vi "Add Module To Project.vi"(6 "TreeControl in":refnum<vi>, 7 "Data Cluster In":T1, 8 "error in":errorcluster) -> (0 "error out":errorcluster, 5 "Data Cluster Out":T1={"DQMH Scan Results"={"All DQMH Modules Refs"=[], "All Modules Descriptions"=[], "All Modules type"=[], "Project References"={"Project Ref"=refnum, "Project Name"="", "App Ref"=refnum, "Target"=refnum, "Target Name"=""}, "Dependencies"=[]}, "Current Selection"={"VI Ref"=refnum, "DQMH Lib Ref"=refnum}, "Module type"=enum."Singleton", "Module ID"=-1, "Theme"=FALSE, "Broadcast?"=FALSE, "Tree Selection"="", "Tree Map"={}})   [LabVIEW 2019, in "Panther Dashboard.lvlib"]
doc: "Gets the Singleton and Cloneable references and creates a list of each type of DQMH Modules"
uses:
  Panther Dashboard.lvlib
  Module Data--cluster.ctl
  DQMH Modules Info--cluster.ctl
  Module type--enum.ctl
  Project References--cluster.ctl
  <vilib>/National Instruments/Tree Map/Tree Map Data.ctl
  <vilib>/National Instruments/Tree Map/API/List Roots.vi
  <vilib>/National Instruments/Tree Map/Utility/Into Tree Control Items.vi
  <vilib>/Delacor/Delacor QMH/Libraries/Scripting API/DQMH_Scripting API.lvlib
  <vilib>/National Instruments/Tree Map/Tree Map.lvlib
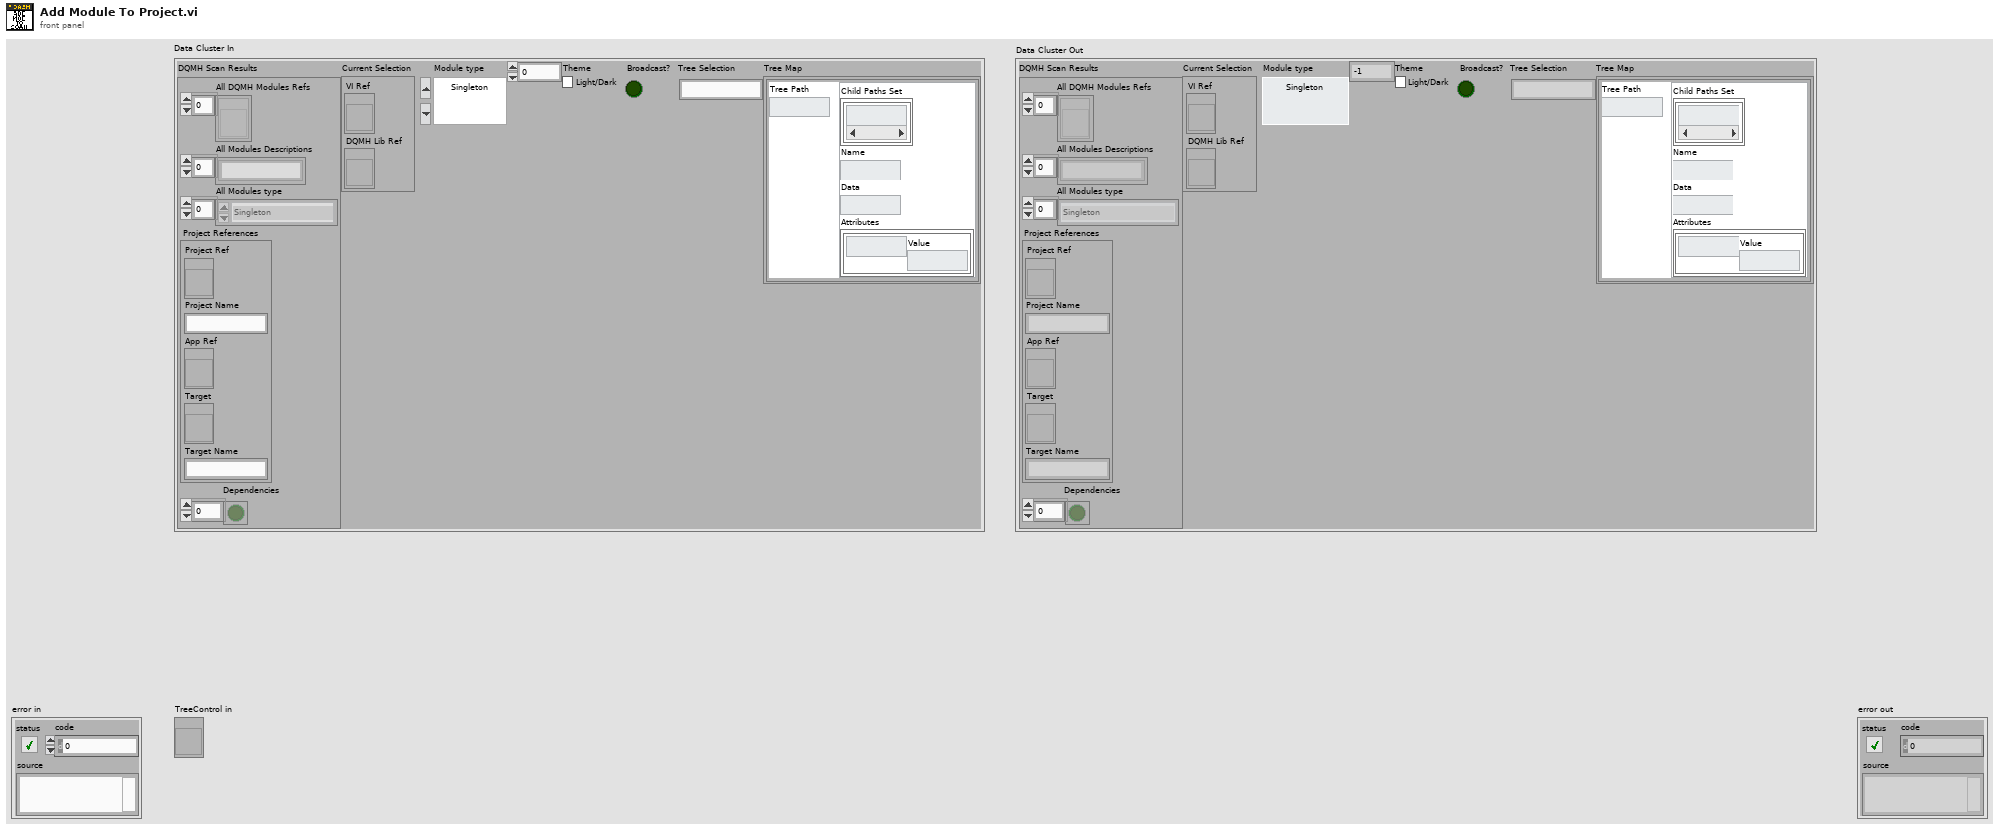
[diagram p1: front panel]
types:
  T1 = typedef "Panther Dashboard.lvlib/Module Data--cluster.ctl" = cluster{"DQMH Scan Results":T2, "Current Selection":cluster{"VI Ref":refnum<vi>, "DQMH Lib Ref":refnum<vi>}, "Module type":T3, "Module ID":i32, "Theme":bool, "Broadcast?":bool, "Tree Selection":string, "Tree Map":T5}
  T2 = typedef "Panther Dashboard.lvlib/DQMH Modules Info--cluster.ctl" = cluster{"All DQMH Modules Refs":refnum<vi>[], "All Modules Descriptions":string[], "All Modules type":T3[], "Project References":T4, "Dependencies":bool[]}
  T3 = typedef "Panther Dashboard.lvlib/Module type--enum.ctl" = enum16{"Singleton", "Cloneable"}
  T4 = typedef "Panther Dashboard.lvlib/Project References--cluster.ctl" = cluster{"Project Ref":refnum<vi>, "Project Name":string, "App Ref":refnum<vi>, "Target":refnum<vi>, "Target Name":string}
  T5 = typedef "Tree Map.lvlib/Tree Map Data.ctl" = map{string, cluster{"Child Paths Set":set{string}, "Name":string, "Data":string, "Attributes":map{string, string}}}
  T6 = typedef "DQMH_Scripting API.lvlib/Module Information--cluster.ctl" = cluster{"Library":refnum<vi>, "Qualified Name":string, "Path":path, "Cloneable":bool, "Under Dependencies":bool}
  T7 = cluster{"Left Cell String":string, "Child Text":string[], "Child Tag":string, "Item Indent":i32, "Child Only?":bool, "Glyph Index":i32}[]
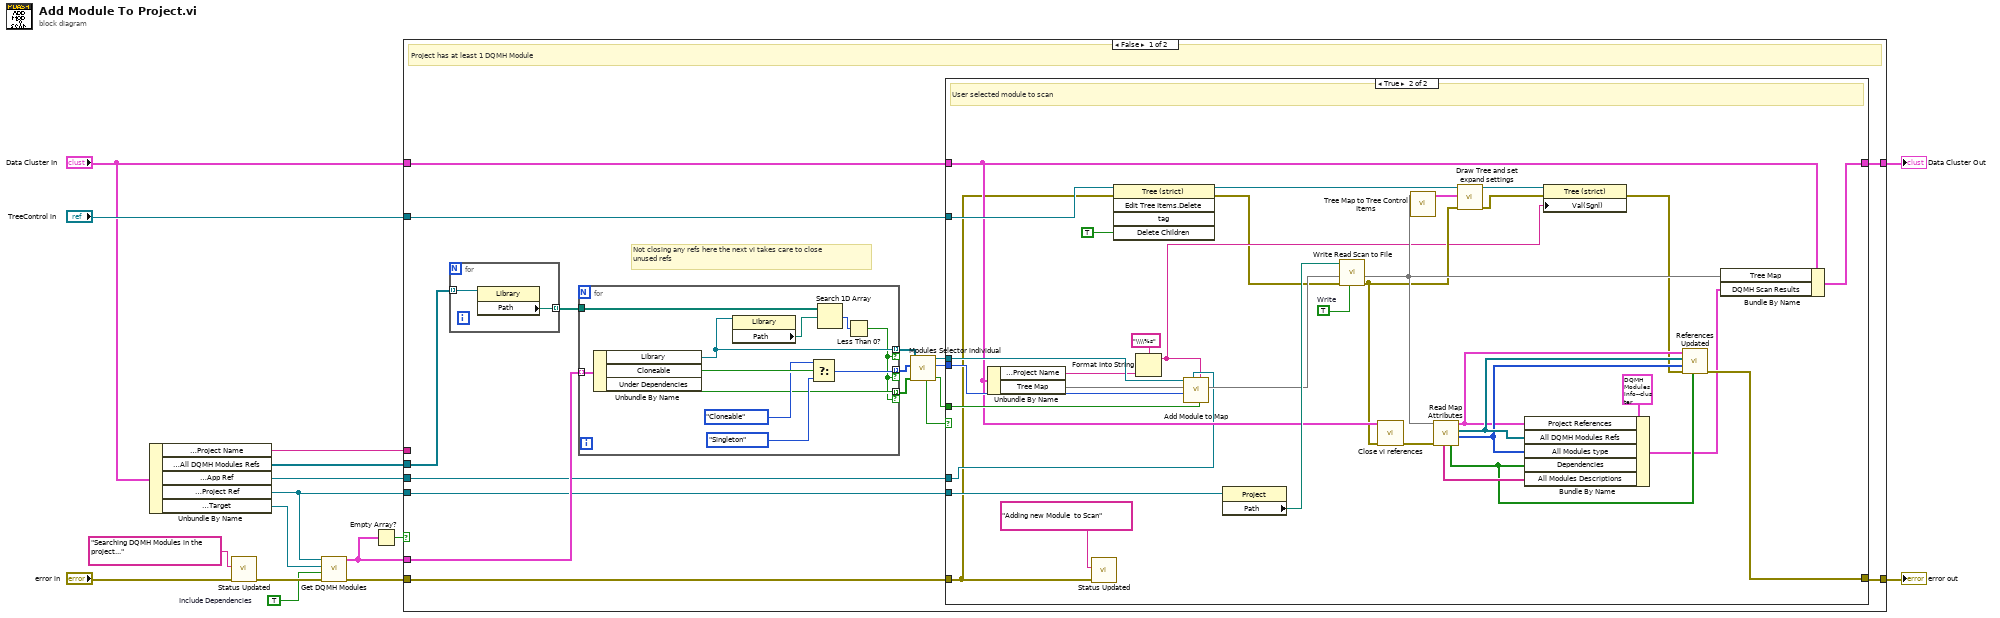
[diagram p0: block diagram]
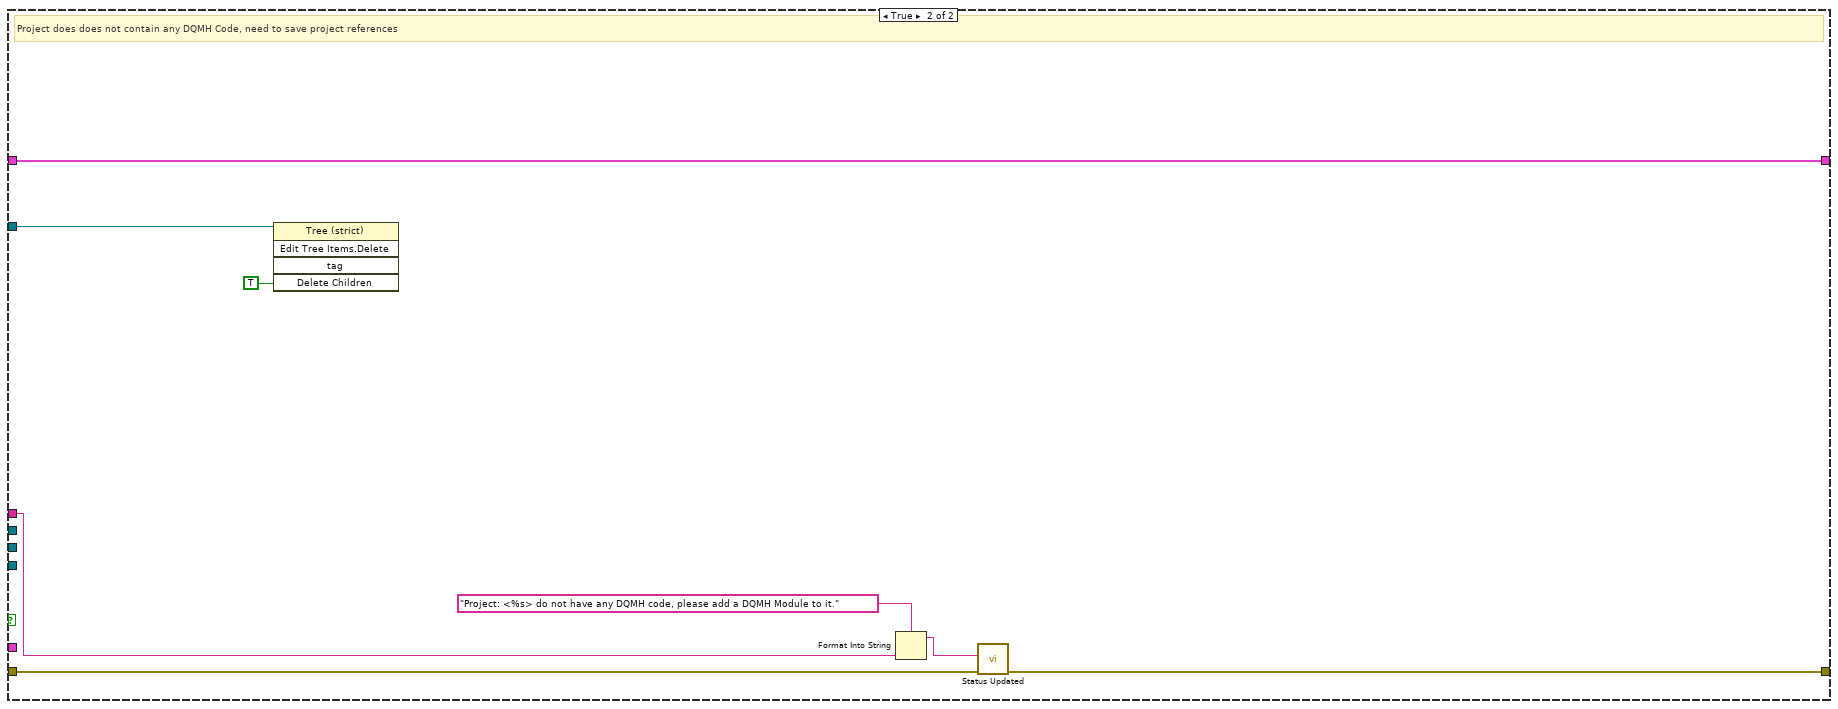
[diagram p3: hidden frame]
diagram:
  w7 = TRUE  # Include Dependencies
  n1 = Unbundle By Name("Data Cluster In") -> ("DQMH Scan Results.Project References.Project Name"=w1:string, "DQMH Scan Results.All DQMH Modules Refs"=w2:refnum<vi>[], "DQMH Scan Results.Project References.App Ref"=w4:refnum<vi>, "DQMH Scan Results.Project References.Project Ref"=w3:refnum<vi>, "DQMH Scan Results.Project References.Target"=w5:refnum<vi>)
  n2 = call "Status Updated.vi"("error in (no error)"="error in", "Status"="Searching DQMH Modules in the project...") -> ("error out"=w14:errorcluster)  [unwired: 9 in]
  n3 = call <vilib>:"Get DQMH Modules.vi"("error in"=w14, "Include Dependencies (F)"=w7, "Target (My Computer)"=w5, "Project"=w3) -> ("error out"=w13:errorcluster, "DQMH Modules"=w8:T6[])  [unwired: 6 in]
  n4 = Empty Array?(array=w8) -> (empty?=w9:bool)
  n5 = case shown="False" w9 {
    tunnel: w13 -> [w33 w91]
    tunnel: [w32 w90] -> w15
    tunnel: "Data Cluster In" -> [w28 w89]
    tunnel: [w27 w89] -> w12
    tunnel: "TreeControl in" -> [w25 w85]
    tunnel: w8 -> [w24 _]
    tunnel: w4 -> [w20 _]
    tunnel: w3 -> [w19 _]
    tunnel: w2 -> [w18 _]
    tunnel: w1 -> [_ w84]
    frame False {
      # "Not closing any refs here the next vi takes care to close \nunused refs"
      # "Project has at least 1 DQMH Module"
      n6 = for {
        tunnel: w18 -> [w83] mode=indexing
        tunnel: [w82] -> w17 mode=indexing
        n7 = property class="Library"(reference=w83) -> ("Path"=w82:path)  [unwired: 1 in, 2 out]
      }
      n8 = for {
        tunnel: w24 -> [w81] mode=indexing
        tunnel: [w74] -> w23 mode=indexing if=w71
        tunnel: [w77] -> w22 mode=indexing if=w71
        tunnel: [w76] -> w21 mode=indexing if=w71
        tunnel: w17 -> [w75]
        n9 = Unbundle By Name(w81) -> ("Library"=w74:refnum<vi>, "Cloneable"=w79:bool, "Under Dependencies"=w76:bool)
        n10 = property class="Library"(reference=w74) -> ("Path"=w73:path)  [unwired: 1 in, 2 out]
        n11 = Select(t=Module_type--enum."Cloneable", s=w79, f=Module_type--enum."Singleton" ("Module type")) -> (s? t:f=w77:T3)
        n12 = Search 1D Array(1D array=w75, element=w73) -> (index of element=w72:i32)  [unwired: 1 in]
        n13 = Less Than 0?(x=w72) -> (x < 0?=w71:bool)
      }
      n14 = call "Modules Selector individual.vi"("Module In Dependencies? in"=w21, "Modules Types In"=w22, "DQMH Modules In"=w23) -> ("Module In Dependencies? Out"=w29:bool, "Modules Type Out"=w31:T3, "DQMH Module Out"=w30:refnum<vi>, "Scan?"=w26:bool)  [unwired: 5 in]
      n15 = case shown="True" w26 {
        tunnel: w31 -> [_ w62]
        tunnel: w30 -> [_ w63]
        tunnel: w29 -> [_ w59]
        tunnel: w28 -> [w34 w58]
        tunnel: [w34 w69] -> w27
        tunnel: w25 -> [_ w67]
        tunnel: w33 -> [w35 w44]
        tunnel: [w35 w70] -> w32
        tunnel: w20 -> [_ w47]
        tunnel: w19 -> [_ w46]
        frame False {
          # "User Cancel Scan process, do not redraw tree and keep previous selection"
        }
        frame True {
          w64 = TRUE  # Write
          # "User selected module to scan"
          n16 = Unbundle By Name(w58) -> ("DQMH Scan Results.Project References.Project Name"=w45:string, "Tree Map"=w61:T5)
          n17 = call "Status Updated.vi"("error in (no error)"=w44, "Status"="Adding new Module  to Scan") -> ()  [unwired: 9 in, 1 out]
          n18 = invoke class="Tree (strict)" method="Edit Tree Items.Delete"(reference=w67, error in=w44, "Delete Children"=TRUE ("Delete Children?")) -> (reference out=w39:refnum<vi>, error out=w40:errorcluster)  [unwired: 2 in, 3 out]
          n19 = Format Into String(format string="\\\\%s", w45) -> (resulting string=w41:string)  [unwired: 2 in, 1 out]
          n20 = call "Add Module to Map.vi"("is Dependency?"=w59, "Parent Path"=w41, "App Ref"=w47, "Module Type"=w62, "Tree Map in"=w61, "Library in"=w63) -> ("Tree Map out"=w60:T5)  [unwired: 4 in, 1 out]
          n21 = property class="Project"(reference=w46) -> ("Path"=w65:path)  [unwired: 1 in, 2 out]
          n22 = call "Write Read Scan to File.vi"("Write"=w64, "error in"=w40, "Tree Map in"=w60, "Path"=w65) -> ("error out"=w42:errorcluster, "Tree Map Out"=w50:T5)  [unwired: 5 in, 1 out]
          n23 = call "Close vi references.vi"("error in"=w42, "Data Cluster"=w58) -> ("error out"=w43:errorcluster)  [unwired: 9 in]
          n24 = call <vilib>:"Tree Map to Tree Control Items.vi"("Tree Map In"=w50) -> ("Tree Control Items"=w68:T7)  [unwired: 10 in]
          n25 = call "Read Map Attributes.vi"("error in"=w43, "Tree Map In (empty)"=w50) -> ("Modules Types Out"=w54:T3[], "Library References"=w57:refnum<vi>[], "References"=w53:T4, "Dependencies?"=w52:bool[], "Descriptions"=w55:string[])  [unwired: 4 in, 1 out]
          n26 = call "Draw Tree and set expand settings.vi"("error in"=w42, "Tree Control Items"=w68, "TreeControl in"=w39) -> ("error out"=w37:errorcluster, "TreeControl out"=w38:refnum<vi>)  [unwired: 7 in]
          n27 = Bundle By Name(cluster=T2 {"All DQMH Modules Refs"=[], "All Modules Descriptions"=[], "All Modules type"=[], "Project References"={"Project Ref"=refnum, "Project Name"="", "App Ref"=refnum, "Target"=refnum, "Target Name"=""}, "Dependencies"=[]} ("DQMH Scan Results"), "Project References"=w53, "All DQMH Modules Refs"=w57, "All Modules type"=w54, "Dependencies"=w52, "All Modules Descriptions"=w55) -> (w51:T2)
          n28 = property class="Tree (strict)"(reference=w38, error in=w37, "Val(Sgnl)"=w41) -> (error out=w36:errorcluster)  [unwired: 1 out]
          n29 = call "References Updated.vi"("Dependencies"=w52, "error in"=w36, "Modules Types"=w54, "Modules"=w57, "References"=w53) -> ("error out"=w70:errorcluster)  [unwired: 6 in]
          n30 = Bundle By Name(cluster=w58, "Tree Map"=w50, "DQMH Scan Results"=w51) -> (w69:T1)
        }
      }
    }
    frame True {
      # "Project does does not contain any DQMH Code, need to save project references"
      n31 = invoke class="Tree (strict)" method="Edit Tree Items.Delete"(reference=w85, "Delete Children"=TRUE ("Delete Children?")) -> ()  [unwired: 3 in, 5 out]
      n32 = Format Into String(format string="Project: <%s> do not have any DQMH code, please add a DQMH Module to it.", w84) -> (resulting string=w88:string)  [unwired: 2 in, 1 out]
      n33 = call "Status Updated.vi"("error in (no error)"=w91, "Status"=w88) -> ("error out"=w90:errorcluster)  [unwired: 9 in]
    }
  }
  "error out" <- w15
  "Data Cluster Out" <- w12
